vi "Calculate Packet Delay Cycles.vi"(8 "current packet  index":i32, 9 "line blanking (cycles)":u64, 10 "minimum delay between packets (cycles)":u64, 11 "packet data types":T1[](array[typedef])) -> (3 "packet delay (cycles)":u64)   [LabVIEW 2023, in "GettingStarted_Gen_148X_Host.lvlib"]
uses:
  GettingStarted_Gen_148X_Host.lvlib
  <instrlib>/FlexRIO/CSI-2/v2/Common/Types/LLP Data Type.ctl
  <instrlib>/FlexRIO/CSI-2/v2/Common/NI CSI-2 API Common v2.lvlib
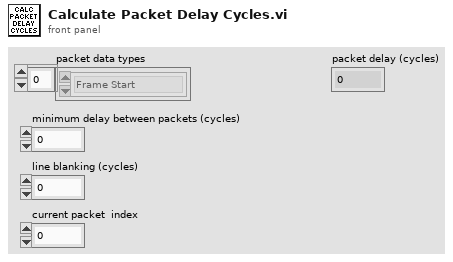
[diagram p1: front panel]
types:
  T1 = typedef "NI CSI-2 API Common v2.lvlib/LLP Data Type.ctl" = enum8{"Frame Start", "Frame End", "Line Start", "Line End", "End of Transmission", "Reserved 0", "Reserved 1", "Reserved 2", "Generic Short Packet 1", "Generic Short Packet 2", "Generic Short Packet 3", "Generic Short Packet 4", "Generic Short Packet 5", "Generic Short Packet 6", "Generic Short Packet 7", "Generic Short Packet 8", "Null", "Blanking Data", "Embedded 8-bit non Image Data", "Generic Long Packet 1", "Generic Long Packet 2", "Generic Long Packet 3", "Generic Long Packet 4", "Reserved 3", "YUV420 8-bit", "YUV420 10-bit", "Legacy YUV420 8-bit", "Reserved 4", "YUV420 8-bit Chroma Shifted", "YUV420 10-bit Chroma Shifted", "YUV422 8-bit", "YUV422 10-bit", "RGB444", "RGB555", "RGB565", "RGB666", "RGB888", "Reserved 5", "Reserved 6", "RAW 24", "RAW 6", "RAW 7", "RAW 8", "RAW 10", "RAW 12", "RAW 14", "RAW 16", "RAW 20", "User Defined 8-bit Data 1", "User Defined 8-bit Data 2", "User Defined 8-bit Data 3", "User Defined 8-bit Data 4", "User Defined 8-bit Data 5", "User Defined 8-bit Data 6", "User Defined 8-bit Data 7", "User Defined 8-bit Data 8", "USL Command", "Reserved 7", "Reserved 8", "Reserved 9", "Reserved 10", "Reserved 11", "Reserved 12", "LRTE EPD Spacer"}
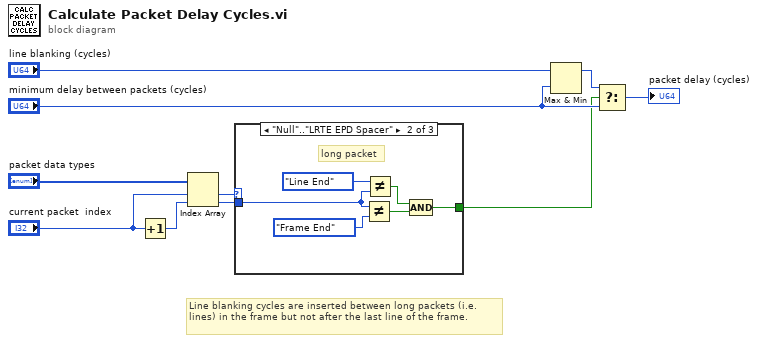
[diagram p0: block diagram]
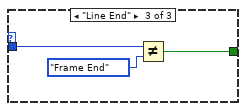
[diagram p3: hidden frame]
diagram:
  # "Line blanking cycles are inserted between long packets (i.e. lines) in the frame but not after the last line of the frame."
  n1 = Increment(x="current packet  index") -> (x+1=w9:i32)
  n2 = Index Array(array="packet data types", index #1="current packet  index", index #2=w9) -> (element #1=w3:T1, element #2=w2:T1)
  n3 = case shown="\"Null\"..\"LRTE EPD Spacer\"" w3 {
    tunnel: w2 -> [_ w15 w19]
    tunnel: [_ w11 w17] -> w1
    frame Default {
    }
    frame "Null".."LRTE EPD Spacer" {
      # "long packet"
      n4 = Not Equal?(x=w15, y=LLP_Data_Type."Frame End" ("element")) -> (x != y?=w12:bool)
      n5 = Not Equal?(x=LLP_Data_Type."Line End", y=w15) -> (x != y?=w13:bool)
      n6 = Compound Arithmetic op=AND(w13, w12) -> (w11:bool)
    }
    frame "Line End" {
      n7 = Not Equal?(x=w19, y=LLP_Data_Type."Frame End" ("element")) -> (x != y?=w17:bool)
    }
  }
  n8 = Max & Min(x="line blanking (cycles)", y="minimum delay between packets (cycles)") -> (max(x,y)=w5:u64)  [unwired: 1 out]
  n9 = Select(t=w5, s=w1, f="minimum delay between packets (cycles)") -> (s? t:f=→"packet delay (cycles)":u64)
